vi "Autonomous Independent.vi"   [LabVIEW 2017]
doc: "This VI is called when autonomous begins, and will automatically be terminated when autonomous ends. You can carry out timed or sensor driven robot movement independently without needing to return to the caller."
uses:
  <vilib>/Rock Robotics/WPI/Utilities/WPI_GetSetVariantRefNum.vi
  <vilib>/Rock Robotics/Network Tables/NT Write Numeric Array.vi
  Robot Global Data.vi
  <vilib>/Rock Robotics/Network Tables/NT Write Number.vi
  <vilib>/Rock Robotics/Network Tables/NT Write String.vi
  <vilib>/Rock Robotics/Network Tables/NT Read String.vi
panel:
  # "Be sure to right-click and choose Data Operations>>Make Current Value default if you want to save the array values with the VI"
types:
  T1 = typedef "WPI_JoystickDevRef.ctl" = cluster{"Device":T2}
  T2 = typedef "WPI_JoystickDeviceEnum.ctl" = enum16{"USB 0", "USB 1", "USB 2", "USB 3", "USB 4", "USB 5"}
  T3 = typedef "WPI_MotorControlDeviceRef.ctl" = cluster{"DeviceStatus":errorcluster, "Type":T4, "PWM":cluster{"PWM Channel":T5, "DeadBand":T6}, "CAN":cluster{"Device Number":u8, "SetOutput VI Ref":variant, "GetOutput VI Ref":variant, "Enable VI Ref":variant, "Disable VI Ref":variant, "Data":variant}, "Invert":bool, "DIO PWM":cluster{"PWM \"Enable\" Channel":T5, "DIOChannel":T7, "PWM Rate":dbl}}
  T4 = typedef "WPI_MotorControlType.ctl" = enum16{"PWM", "CAN", "DIO PWM"}
  T5 = typedef "FPGA_DIOPWMChannel.ctl" = enum8{"PWM 0", "PWM 1", "PWM 2", "PWM 3", "PWM 4", "PWM 5", "PWM 6", "PWM 7", "PWM 8", "PWM 9", "PWM MXP 0", "PWM MXP 1", "PWM MXP 2", "PWM MXP 3", "PWM MXP 4", "PWM MXP 5", "PWM MXP 6", "PWM MXP 7", "PWM MXP 8", "PWM MXP 9", "Invalid"}
  T6 = typedef "WPI_PWMDeadband.ctl" = cluster{"Name":string, "maxPositivePwm":i32, "minPositivePwm":i32, "centerPwm":i32, "maxNegativePwm":i32, "minNegativePwm":i32, "angularRange":u16}
  T7 = typedef "FPGA_DIOChannel.ctl" = enum8{"DIO 0", "DIO 1", "DIO 2", "DIO 3", "DIO 4", "DIO 5", "DIO 6", "DIO 7", "DIO 8", "DIO 9", "DIO MXP 0", "DIO MXP 1", "DIO MXP 2", "DIO MXP 3", "DIO MXP 4", "DIO MXP 5", "DIO MXP 6", "DIO MXP 7", "DIO MXP 8", "DIO MXP 9", "DIO MXP 10", "DIO MXP 11", "DIO MXP 12", "DIO MXP 13", "DIO MXP 14", "DIO MXP 15", "SPI Port CS1", "SPI Port CS2", "SPI Port CS3", "SPI Port MISO", "SPI Port MOSI", "Invalid"}
  T8 = typedef "WPI_DigitalInputDevRef.ctl" = cluster{"DevStatus":errorcluster, "DIO Channel":T7}
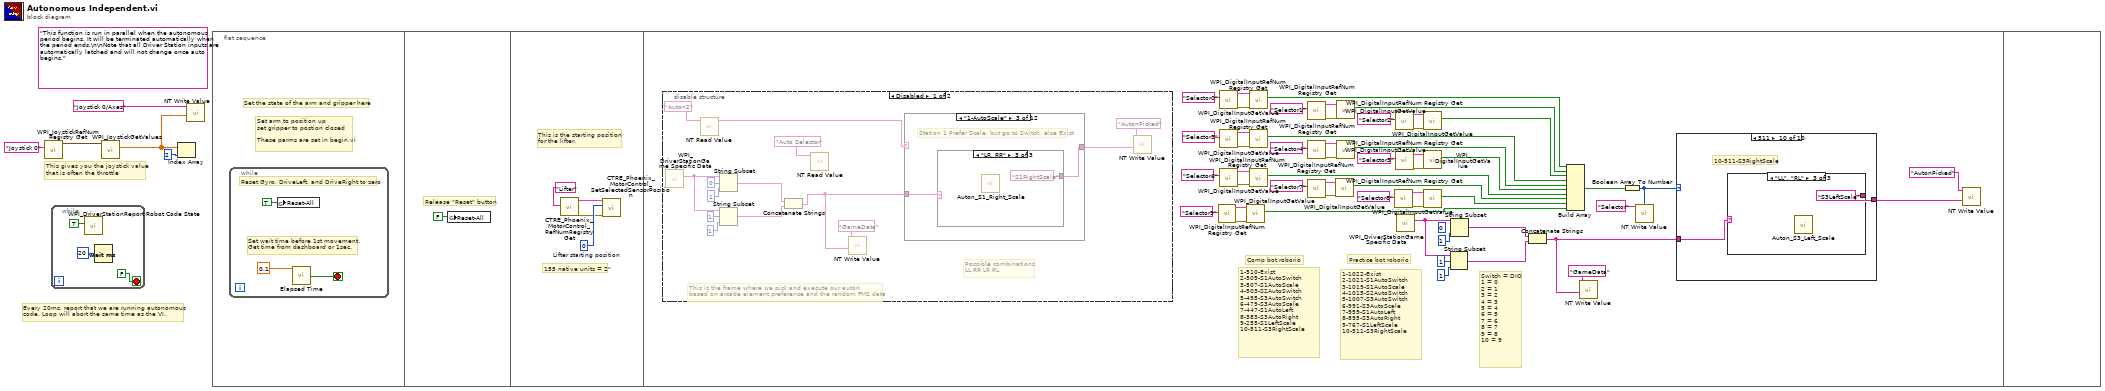
[diagram p0: block diagram]
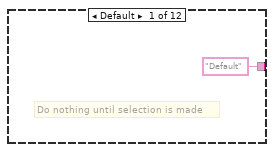
[diagram p2: hidden frame]
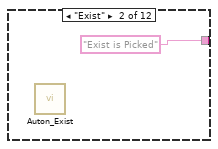
[diagram p3: hidden frame]
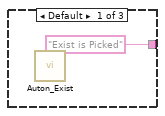
[diagram p4: hidden frame]
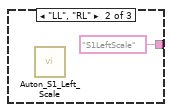
[diagram p5: hidden frame]
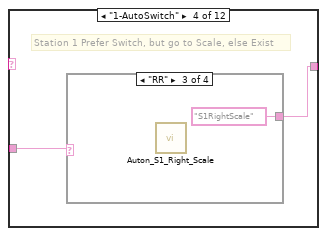
[diagram p6: hidden frame]
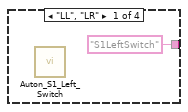
[diagram p7: hidden frame]
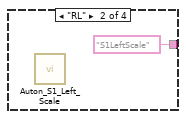
[diagram p8: hidden frame]
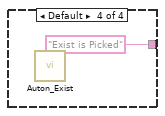
[diagram p9: hidden frame]
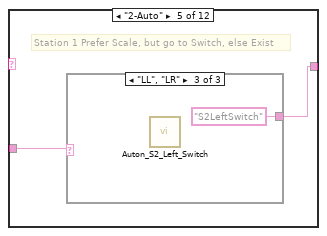
[diagram p10: hidden frame]
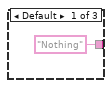
[diagram p11: hidden frame]
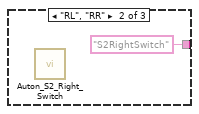
[diagram p12: hidden frame]
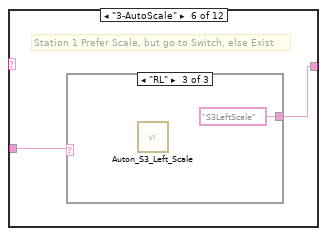
[diagram p13: hidden frame]
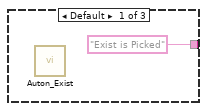
[diagram p14: hidden frame]
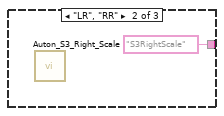
[diagram p15: hidden frame]
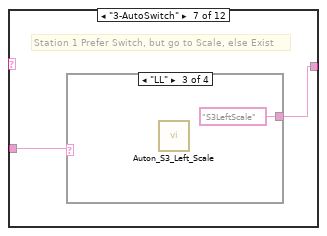
[diagram p16: hidden frame]
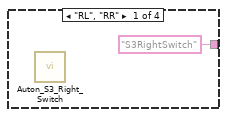
[diagram p17: hidden frame]
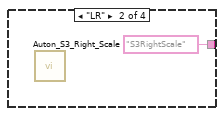
[diagram p18: hidden frame]
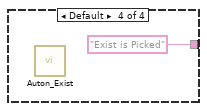
[diagram p19: hidden frame]
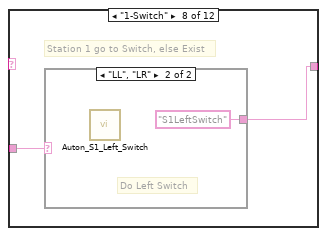
[diagram p20: hidden frame]
diagram:
  (unwired) "This function is run in parallel when the autonomous period begins. It will be terminated automatically when the period ends.\n\nNote that all Driver Station inputs are automatically latched and will not change once auto begins."
  # "Every 20ms, report that we are running autonomous\ncode. Loop will abort the same time as the VI."
  # "This gives you the joystick value\nthat is often the throttle"
  n1 = call <vilib>:"WPI_JoystickRefNum Registry Get.vi"("refnum name"="Joystick 0") -> ("JoystickDevRef"=w4:T1)  [unwired: 1 in, 9 out]
  n2 = while {
    stop <- FALSE stop-if-true
    n3 = call <vilib>:"WPI_DriverStationReport Robot Code State.vi"("Autonomous"=TRUE) -> ()  [unwired: 10 in, 1 out]
    n4 = Wait (ms)(milliseconds to wait=u32 20) -> ()  [unwired: 1 out]
  }
  n5 = call <vilib>:"WPI_JoystickGetValues.vi"("JoystickDevRef"=w4) -> ("Axes"=w2:dbl[])  [unwired: 6 in, 4 out]
  n6 = Index Array(array=w2, index=2) -> ()  [unwired: 1 out]
  n7 = call-poly <vilib>:"NT Write Value.vi"("Numeric Array"=w2, "Name"="Joystick 0/Axes") -> ()  [unwired: 9 in, 1 out]
  n8 = flat-sequence {
    frame #0 {
      # "Set arm to position up\nset gripper to postion closed\n\nThese parms are set in begin.vi"
      # "Set the state of the arm and gripper here"
      n9 = while {
        stop <- w11 stop-if-true
        # "Set wait time before 1st movement.\nGet time from dashboard or 1sec."
        # "Reset Gyro, DriveLeft, and DriveRight to zero"
        n10 = global write "Robot Global Data.vi" "Reset-All"(TRUE ("Reset")) -> ()
        n11 = call "Elapsed Time"("Time Target (s)"=0.1) -> ("Time has Elapsed"=w11:bool)  [unwired: 11 in, 7 out]
      }
    }
    frame #1 {
      # "Release \"Reset\" button"
      n12 = global write "Robot Global Data.vi" "Reset-All"(FALSE ("Reset")) -> ()
    }
    frame #2 {
      w16 = 0  # Lifter starting position
      # "This is the starting position\nfor the lifter."
      # "155 native units = 2\""
      n13 = call <vilib>:"CTRE_Phoenix_MotorControl_RefNumRegistryGet.vi"("refnum name"="Lifter") -> ("error out"=w14:errorcluster, "PhoenixMotorControlDevRef"=w15:T3)  [unwired: 9 in]
      n14 = call <vilib>:"CTRE_Phoenix_MotorControl_SetSelectedSensorPosition.vi"("error in (no error)"=w14, "New Sensor Position"=w16, "PhoenixMotorControlDevRef"=w15) -> ()  [unwired: 7 in, 2 out]
    }
    frame #3 {
      (unwired) 0 ("offset (0)")
      # "Switch = DIO\n1 = 0\n2 = 1\n3 = 2\n4 = 3\n5 = 4\n6 = 5\n7 = 6\n8 = 7\n9 = 8\n10 = 9"
      # "1-1022-Exist\n2-1021-S1AutoSwitch\n3-1019-S1AutoScale\n4-1015-S2AutoSwitch\n5-1007-S3AutoSwitch\n6-991-S3AutoScale\n7-959-S1AutoLeft\n8-895-S3AutoRight\n9-767-S1LeftScale\n10-511-S3RightScale"
      # "Practice bot roborio"
      # "Comp bot roborio"
      # "1-510-Exist\n2-509-S1AutoSwitch\n3-507-S1AutoScale\n4-503-S2AutoSwitch\n5-495-S3AutoSwitch\n6-479-S3AutoScale\n7-447-S1AutoLeft\n8-383-S3AutoRight\n9-255-S1LeftScale\n10-511-S3RightScale"
      n15 = disable-structure shown="Disabled" {
        frame Disabled {
          # "Possible combinations\nLL RR LR RL"
          # "This is the frame where we pick and execute our auton\nbased on arcade element preference and the random FMS data"
          n16 = call <vilib>:"WPI_DriverStationGame Specific Data.vi"() -> ("Game Specific Data"=w80:string)  [unwired: 11 in]
          n17 = call-poly <vilib>:"NT Read Value.vi"("Name"="Auton2") -> ("String"=w70:string)  [unwired: 9 in, 1 out]
          n18 = String Subset(string=w80, offset (0)=1, length (rest)=1 ("length (rest)")) -> (substring=w77:string)
          n19 = String Subset(string=w80, offset (0)=0, length (rest)=1 ("length (rest)")) -> (substring=w76:string)
          n20 = Concatenate Strings(w76, w77) -> (w74:string)
          n21 = call-poly <vilib>:"NT Read Value.vi"("Name"="Auto Selector") -> ()  [unwired: 9 in, 2 out]
          n22 = call-poly <vilib>:"NT Write Value.vi"("String"=w74, "Name"="GameData") -> ()  [unwired: 9 in, 1 out]
          n23 = case shown="\"1-AutoScale\"" w70 {
            tunnel: w74 -> [_ _ w87 w92 w98 w103 w108 w114 w118 w122 w126 _]
            tunnel: ["Default" "Exist is Picked" w86 w91 w97 w102 w107 w113 w117 w121 w125 "MiniExist"] -> w73
            frame Default {
              # "Do nothing until selection is made"
            }
            frame "Exist" {
              n24 = call "Auton_Exist.vi"() -> ()  [unwired: 12 in]
            }
            frame "1-AutoScale" {
              # "Station 1 Prefer Scale, but go to Switch, else Exist"
              n25 = case shown="\"LR, RR\"" w87 {
                tunnel: ["Exist is Picked" "S1LeftScale" "S1RightScale"] -> w86
                frame Default {
                  n26 = call "Auton_Exist.vi"() -> ()  [unwired: 12 in]
                }
                frame "LL", "RL" {
                  n27 = call "Auton_S1_Left_Scale.vi"() -> ()  [unwired: 12 in]
                }
                frame "LR, RR" {
                  n28 = call "Auton_S1_Right_Scale.vi"() -> ()  [unwired: 12 in]
                }
              }
            }
            frame "1-AutoSwitch" {
              # "Station 1 Prefer Switch, but go to Scale, else Exist"
              n29 = case shown="\"RR\"" w92 {
                tunnel: ["S1LeftSwitch" "S1LeftScale" "S1RightScale" "Exist is Picked"] -> w91
                frame "LL", "LR" {
                  n30 = call "Auton_S1_Left_Switch.vi"() -> ()  [unwired: 12 in]
                }
                frame "RL" {
                  n31 = call "Auton_S1_Left_Scale.vi"() -> ()  [unwired: 12 in]
                }
                frame "RR" {
                  n32 = call "Auton_S1_Right_Scale.vi"() -> ()  [unwired: 12 in]
                }
                frame Default {
                  n33 = call "Auton_Exist.vi"() -> ()  [unwired: 12 in]
                }
              }
            }
            frame "2-Auto" {
              # "Station 1 Prefer Scale, but go to Switch, else Exist"
              n34 = case shown="\"LL\", \"LR\"" w98 {
                tunnel: ["Nothing" "S2RightSwitch" "S2LeftSwitch"] -> w97
                frame Default {
                }
                frame "RL", "RR" {
                  n35 = call "Auton_S2_Right_Switch.vi"() -> ()  [unwired: 12 in]
                }
                frame "LL", "LR" {
                  n36 = call "Auton_S2_Left_Switch.vi"() -> ()  [unwired: 12 in]
                }
              }
            }
            frame "3-AutoScale" {
              # "Station 1 Prefer Scale, but go to Switch, else Exist"
              n37 = case shown="\"RL\"" w103 {
                tunnel: ["Exist is Picked" "S3RightScale" "S3LeftScale"] -> w102
                frame Default {
                  n38 = call "Auton_Exist.vi"() -> ()  [unwired: 12 in]
                }
                frame "LR", "RR" {
                  n39 = call "Auton_S3_Right_Scale.vi"() -> ()  [unwired: 12 in]
                }
                frame "RL" {
                  n40 = call "Auton_S3_Left_Scale.vi"() -> ()  [unwired: 12 in]
                }
              }
            }
            frame "3-AutoSwitch" {
              # "Station 1 Prefer Switch, but go to Scale, else Exist"
              n41 = case shown="\"LL\"" w108 {
                tunnel: ["S3RightSwitch" "S3RightScale" "S3LeftScale" "Exist is Picked"] -> w107
                frame "RL", "RR" {
                  n42 = call "Auton_S3_Right_Switch.vi"() -> ()  [unwired: 12 in]
                }
                frame "LR" {
                  n43 = call "Auton_S3_Right_Scale.vi"() -> ()  [unwired: 12 in]
                }
                frame "LL" {
                  n44 = call "Auton_S3_Left_Scale.vi"() -> ()  [unwired: 12 in]
                }
                frame Default {
                  n45 = call "Auton_Exist.vi"() -> ()  [unwired: 12 in]
                }
              }
            }
            frame "1-Switch" {
              # "Station 1 go to Switch, else Exist"
              n46 = case shown="\"LL\", \"LR\"" w114 {
                tunnel: ["Exist is Picked" "S1LeftSwitch"] -> w113
                frame Default {
                  # "Do Exist"
                  n47 = call "Auton_Exist.vi"() -> ()  [unwired: 12 in]
                }
                frame "LL", "LR" {
                  # "Do Left Switch"
                  n48 = call "Auton_S1_Left_Switch.vi"() -> ()  [unwired: 12 in]
                }
              }
            }
            frame "1-Scale" {
              # "Station 1 go to Scale, else Exist"
              n49 = case shown="\"LL\", \"RL\"" w118 {
                tunnel: ["Exist is Picked" "S1LeftScale"] -> w117
                frame Default {
                  # "Do Exist"
                  n50 = call "Auton_Exist.vi"() -> ()  [unwired: 12 in]
                }
                frame "LL", "RL" {
                  # "Do Left Scale"
                  n51 = call "Auton_S1_Left_Scale.vi"() -> ()  [unwired: 12 in]
                }
              }
            }
            frame "3-Switch" {
              # "Station 1 go to Switch, else Exist"
              n52 = case shown="\"RL\", \"RR\"" w122 {
                tunnel: ["Exist is Picked" "S3RightSwitch"] -> w121
                frame Default {
                  # "Do Exist"
                  n53 = call "Auton_Exist.vi"() -> ()  [unwired: 12 in]
                }
                frame "RL", "RR" {
                  # "Do Left Switch"
                  n54 = call "Auton_S3_Right_Switch.vi"() -> ()  [unwired: 12 in]
                }
              }
            }
            frame "3-Scale" {
              # "Station 1 go to Scale, else Exist"
              n55 = case shown="\"LR\", \"RR\"" w126 {
                tunnel: ["Exist is Picked" "S3RightScale"] -> w125
                frame Default {
                  # "Do Exist"
                  n56 = call "Auton_Exist.vi"() -> ()  [unwired: 12 in]
                }
                frame "LR", "RR" {
                  # "Do Left Scale"
                  n57 = call "Auton_S3_Right_Scale.vi"() -> ()  [unwired: 12 in]
                }
              }
            }
            frame "MiniExist" {
              n58 = call "Auton_S2_Right_Switch.vi"() -> ()  [unwired: 12 in]
            }
          }
          n59 = call-poly <vilib>:"NT Write Value.vi"("String"=w73, "Name"="AutonPicked") -> ()  [unwired: 9 in, 1 out]
        }
        frame Enabled {
        }
      }
      n60 = call <vilib>:"WPI_DigitalInputRefNum Registry Get.vi"("refnum name"="Selector9") -> ("error out"=w20:errorcluster, "DigitalInputDevRef"=w19:T8)  [unwired: 9 in]
      n61 = call <vilib>:"WPI_DigitalInputRefNum Registry Get.vi"("refnum name"="Selector6") -> ("error out"=w42:errorcluster, "DigitalInputDevRef"=w43:T8)  [unwired: 9 in]
      n62 = call <vilib>:"WPI_DigitalInputRefNum Registry Get.vi"("refnum name"="Selector0") -> ("error out"=w64:errorcluster, "DigitalInputDevRef"=w65:T8)  [unwired: 9 in]
      n63 = call <vilib>:"WPI_DigitalInputRefNum Registry Get.vi"("refnum name"="Selector3") -> ("error out"=w54:errorcluster, "DigitalInputDevRef"=w55:T8)  [unwired: 9 in]
      n64 = call <vilib>:"WPI_DigitalInputGetValue.vi"("error in (no error)"=w20, "DigitalInputDevRef"=w19) -> ("Value"=w17:bool)  [unwired: 7 in, 2 out]
      n65 = call <vilib>:"WPI_DigitalInputGetValue.vi"("error in (no error)"=w42, "DigitalInputDevRef"=w43) -> ("Value"=w37:bool)  [unwired: 7 in, 2 out]
      n66 = call <vilib>:"WPI_DigitalInputGetValue.vi"("error in (no error)"=w64, "DigitalInputDevRef"=w65) -> ("Value"=w33:bool)  [unwired: 7 in, 2 out]
      n67 = call <vilib>:"WPI_DigitalInputGetValue.vi"("error in (no error)"=w54, "DigitalInputDevRef"=w55) -> ("Value"=w49:bool)  [unwired: 7 in, 2 out]
      n68 = call <vilib>:"WPI_DigitalInputRefNum Registry Get.vi"("refnum name"="Selector7") -> ("error out"=w46:errorcluster, "DigitalInputDevRef"=w45:T8)  [unwired: 9 in]
      n69 = call <vilib>:"WPI_DigitalInputRefNum Registry Get.vi"("refnum name"="Selector1") -> ("error out"=w68:errorcluster, "DigitalInputDevRef"=w67:T8)  [unwired: 9 in]
      n70 = call <vilib>:"WPI_DigitalInputRefNum Registry Get.vi"("refnum name"="Selector4") -> ("error out"=w58:errorcluster, "DigitalInputDevRef"=w57:T8)  [unwired: 9 in]
      n71 = call <vilib>:"WPI_DigitalInputGetValue.vi"("error in (no error)"=w46, "DigitalInputDevRef"=w45) -> ("Value"=w36:bool)  [unwired: 7 in, 2 out]
      n72 = call <vilib>:"WPI_DigitalInputGetValue.vi"("error in (no error)"=w68, "DigitalInputDevRef"=w67) -> ("Value"=w69:bool)  [unwired: 7 in, 2 out]
      n73 = call <vilib>:"WPI_DigitalInputGetValue.vi"("error in (no error)"=w58, "DigitalInputDevRef"=w57) -> ("Value"=w48:bool)  [unwired: 7 in, 2 out]
      n74 = call <vilib>:"WPI_DigitalInputRefNum Registry Get.vi"("refnum name"="Selector8") -> ("error out"=w40:errorcluster, "DigitalInputDevRef"=w39:T8)  [unwired: 9 in]
      n75 = call <vilib>:"WPI_DigitalInputRefNum Registry Get.vi"("refnum name"="Selector2") -> ("error out"=w62:errorcluster, "DigitalInputDevRef"=w61:T8)  [unwired: 9 in]
      n76 = call <vilib>:"WPI_DigitalInputRefNum Registry Get.vi"("refnum name"="Selector5") -> ("error out"=w52:errorcluster, "DigitalInputDevRef"=w51:T8)  [unwired: 9 in]
      n77 = call <vilib>:"WPI_DriverStationGame Specific Data.vi"() -> ("Game Specific Data"=w26:string)  [unwired: 11 in]
      n78 = call <vilib>:"WPI_DigitalInputGetValue.vi"("error in (no error)"=w40, "DigitalInputDevRef"=w39) -> ("Value"=w35:bool)  [unwired: 7 in, 2 out]
      n79 = call <vilib>:"WPI_DigitalInputGetValue.vi"("error in (no error)"=w62, "DigitalInputDevRef"=w61) -> ("Value"=w59:bool)  [unwired: 7 in, 2 out]
      n80 = call <vilib>:"WPI_DigitalInputGetValue.vi"("error in (no error)"=w52, "DigitalInputDevRef"=w51) -> ("Value"=w47:bool)  [unwired: 7 in, 2 out]
      n81 = String Subset(string=w26, offset (0)=1, length (rest)=1 ("length (rest)")) -> (substring=w24:string)
      n82 = String Subset(string=w26, length (rest)=1 ("length (rest)")) -> (substring=w23:string)  [unwired: 1 in]
      n83 = Concatenate Strings(w23, w24) -> (w25:string)
      n84 = Build Array(w33, w69, w59, w49, w48, w47, w37, w36, w35, w17) -> (w34:bool[])
      n85 = call-poly <vilib>:"NT Write Value.vi"("String"=w25, "Name"="GameData") -> ()  [unwired: 9 in, 1 out]
      n86 = Boolean Array To Number(Boolean array=w34) -> (number=w22:u32)
      n87 = call-poly <vilib>:"NT Write Value.vi"("Numeric"=w22, "Name"="Selector") -> ()  [unwired: 9 in, 1 out]
      n88 = case shown="511" w22 {
        tunnel: ["Exist is Picked" w132 w139 w144 w149 w156 w161 w167 w173 w178] -> w31
        tunnel: w25 -> [_ w131 w138 w143 w148 w155 w160 w166 w172 w177]
        frame 510, 1022, Default {
          # "s1 - dio 0"
          # "Exist"
          n89 = call "Auton_Exist.vi"() -> ()  [unwired: 12 in]
        }
        frame 509, 1021 {
          # "s2-dio1"
          # "S1Autoswitch"
          n90 = case shown="\"RR\"" w131 {
            tunnel: ["S1LeftSwitch" "S1LeftScale&Switch" "S1LeftScale" "S1RightScale" "Error"] -> w132
            frame "LR" {
              n91 = call "Auton_S1_Left_Switch.vi"() -> ()  [unwired: 12 in]
            }
            frame "LL" {
              n92 = call "Auton_S1_Left_Scale_Left_Switch_2Cube.vi"() -> ()  [unwired: 12 in]
            }
            frame "RL" {
              n93 = call "Auton_S1_Left_Scale.vi"() -> ()  [unwired: 12 in]
            }
            frame "RR" {
              n94 = call "Auton_S1_Right_Scale.vi"() -> ()  [unwired: 12 in]
            }
            frame Default {
              n95 = call "Auton_Exist.vi"() -> ()  [unwired: 12 in]
            }
          }
        }
        frame 507, 1019 {
          # "S1AutoScale"
          n96 = case shown="\"LL\", \"RL\"" w138 {
            tunnel: ["Error" "S1LeftScale2Cube" "S1RightScale"] -> w139
            frame Default {
              n97 = call "Auton_Exist.vi"() -> ()  [unwired: 12 in]
            }
            frame "LL", "RL" {
              n98 = call "Auton_S1_Left_Scale_2Cube.vi"() -> ()  [unwired: 12 in]
            }
            frame "LR", "RR" {
              n99 = call "Auton_S1_Right_Scale.vi"() -> ()  [unwired: 12 in]
            }
          }
        }
        frame 503, 1015 {
          # "S2AutoSwitch"
          n100 = case shown="\"RL\", \"RR\"" w143 {
            tunnel: ["Error" "S2RightSwitch" "S2LeftSwitch"] -> w144
            frame Default {
            }
            frame "RL", "RR" {
              n101 = call "Auton_S2_Right_Switch.vi"() -> ()  [unwired: 12 in]
            }
            frame "LL", "LR" {
              n102 = call "Auton_S2_Left_Switch.vi"() -> ()  [unwired: 12 in]
            }
          }
        }
        frame 495, 1007 {
          # "S3AutoSwitch"
          n103 = case shown="Default" w148 {
            tunnel: ["S3RightSwitch" "S3RightScale&Switch" "S3RightScale" "S3LeftScale" "Error"] -> w149
            frame "RL" {
              n104 = call "Auton_S3_Right_Switch.vi"() -> ()  [unwired: 12 in]
            }
            frame "RR" {
              n105 = call "Auton_S3_Right_Scale_Right_Switch_2Cube.vi"() -> ()  [unwired: 12 in]
            }
            frame "LR" {
              n106 = call "Auton_S3_Right_Scale.vi"() -> ()  [unwired: 12 in]
            }
            frame "LL" {
              n107 = call "Auton_S3_Left_Scale.vi"() -> ()  [unwired: 12 in]
            }
            frame Default {
              n108 = call "Auton_Exist.vi"() -> ()  [unwired: 12 in]
            }
          }
        }
        frame 479, 991 {
          # "S3AutoScale"
          n109 = case shown="\"LL\", \"RL\"" w155 {
            tunnel: ["Error" "S3RightScale2Cube" "S3LeftScale"] -> w156
            frame Default {
              n110 = call "Auton_Exist.vi"() -> ()  [unwired: 12 in]
            }
            frame "LR", "RR" {
              n111 = call "Auton_S3_Right_Scale_2Cube.vi"() -> ()  [unwired: 12 in]
            }
            frame "LL", "RL" {
              n112 = call "Auton_S3_Left_Scale.vi"() -> ()  [unwired: 12 in]
            }
          }
        }
        frame 447, 959 {
          # "7-447-S1AutoLeft"
          n113 = case shown="\"LL\"" w160 {
            tunnel: ["Exist is Picked" "S1LeftScale" "S1LeftScale&Switch" "S1LeftSwitch"] -> w161
            frame Default {
              n114 = call "Auton_Exist.vi"() -> ()  [unwired: 12 in]
            }
            frame "RL" {
              n115 = call "Auton_S1_Left_Scale.vi"() -> ()  [unwired: 12 in]
            }
            frame "LL" {
              n116 = call "Auton_S1_Left_Scale_Left_Switch_2Cube.vi"() -> ()  [unwired: 12 in]
            }
            frame "LR" {
              n117 = call "Auton_S1_Left_Switch.vi"() -> ()  [unwired: 12 in]
            }
          }
        }
        frame 383, 895 {
          # "8-383-S3AutoRight"
          n118 = case shown="\"RR\"" w166 {
            tunnel: ["Exist is Picked" "S3RightScale" "S3RightSwitch" "S3RightScale&Switch"] -> w167
            frame Default {
              n119 = call "Auton_Exist.vi"() -> ()  [unwired: 12 in]
            }
            frame "LR" {
              n120 = call "Auton_S3_Right_Scale.vi"() -> ()  [unwired: 12 in]
            }
            frame "RL" {
              n121 = call "Auton_S3_Right_Switch.vi"() -> ()  [unwired: 12 in]
            }
            frame "RR" {
              n122 = call "Auton_S3_Right_Scale_Right_Switch_2Cube.vi"() -> ()  [unwired: 12 in]
            }
          }
        }
        frame 255, 767 {
          # "9-255-S1OldAutoScale"
          n123 = case shown="\"LR\", \"RR\"" w172 {
            tunnel: ["Exist is Picked" "S1LeftScale" "S3RightScale"] -> w173
            frame Default {
              # "Do Exist"
              n124 = call "Auton_S1_Right_Scale_2Cube.vi"() -> ()  [unwired: 12 in]
            }
            frame "LL", "RL" {
              # "Do Left Scale 2 Cube"
              n125 = call "Auton_S1_Left_Scale.vi"() -> ()  [unwired: 12 in]
            }
            frame "LR", "RR" {
              n126 = call "Auton_S1_Right_Scale.vi"() -> ()  [unwired: 12 in]
            }
          }
        }
        frame 511 {
          # "10-511-S3RightScale"
          n127 = case shown="\"LL\", \"RL\"" w177 {
            tunnel: ["Exist is Picked" "S3RightScale" "S3LeftScale"] -> w178
            frame Default {
              # "Do Exist"
              n128 = call "Auton_Exist.vi"() -> ()  [unwired: 12 in]
            }
            frame "LR", "RR" {
              n129 = call "Auton_S3_Right_Scale.vi"() -> ()  [unwired: 12 in]
            }
            frame "LL", "RL" {
              n130 = call "Auton_S3_Left_Scale.vi"() -> ()  [unwired: 12 in]
            }
          }
        }
      }
      n131 = call-poly <vilib>:"NT Write Value.vi"("String"=w31, "Name"="AutonPicked") -> ()  [unwired: 9 in, 1 out]
    }
    frame #4 {
    }
  }
